vi "NI9472.vi"() -> ()   [LabVIEW 2019]
panel:
  out "7 LED":bool
  in  "DO 7":bool
  out "0 LED":bool
  in  "DO 0":bool
  # "NI 9472 Control"
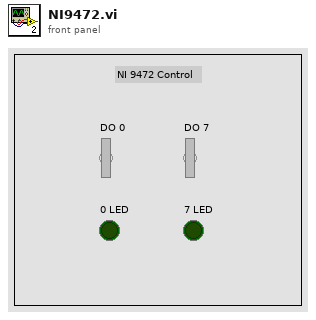
[diagram p1: front panel]
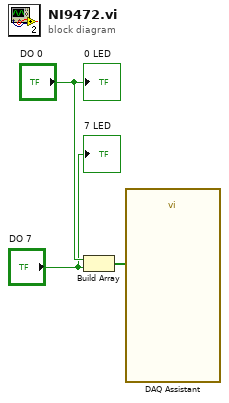
[diagram p0: block diagram]
diagram:
  n1 = Build Array("DO 0", "DO 7") -> (w2:bool[])
  n2 = call "DAQ Assistant"("data"=w2) -> ()  [unwired: 17 in, 2 out]
  "0 LED" <- "DO 0"
  "7 LED" <- "DO 7"
